vi "CLC_JIO_subUDC.vi"(5 "Mode":T1=enum."Tx", 8 "error in":errorcluster, 10 "ud att":i32) -> (0 "error out":errorcluster, 3 "standard output":string)   [LabVIEW 2023, in "CLC_JIO_FTDI.lvlib"]
uses:
  CLC_JIO_FTDI.lvlib
  CTL/Mode_tx1_rx2.ctl
panel:
  out "appended path":path
  out "standard error":string
  out "floder?":bool
  # "0:Tx\n1:Rx"
  # "0-255"
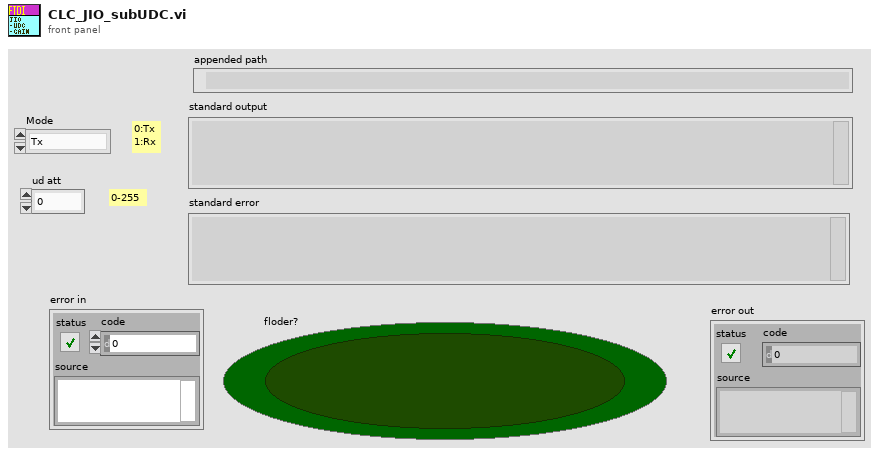
[diagram p1: front panel]
types:
  T1 = typedef "Mode_tx1_rx2.ctl" = enum16{"Standy", "Tx", "Rx"}
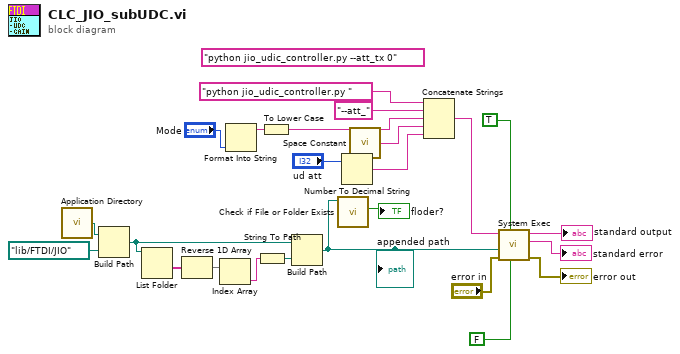
[diagram p0: block diagram]
diagram:
  (unwired) "python jio_udic_controller.py --att_tx 0" ("command line")
  n1 = call <vilib>:"Application Directory.vi"() -> ("Application Directory"=w16:path)
  n2 = Build Path(base path=w16, name or relative path=path "lib/FTDI/JIO") -> (appended path=w15:path)
  n3 = List Folder(path=w15) -> (folder names=w21:string[])  [unwired: 3 in, 3 out]
  n4 = Reverse 1D Array(array=w21) -> (reversed array=w20:string[])
  n5 = Index Array(array=w20) -> (element=w19:string)  [unwired: 1 in]
  n6 = Format Into String("Mode") -> (resulting string=w23:string)  [unwired: 3 in, 1 out]
  n7 = String To Path(string=w19) -> (path=w18:path)
  n8 = To Lower Case(string=w23) -> (all lower case string=w1:string)
  n9 = Build Path(base path=w15, name or relative path=w18) -> (appended path=w13:path)
  "appended path" <- w13
  n10 = call <vilib>:"Check if File or Folder Exists.vi"("path"=w13) -> ("file or folder exists?"=→"floder?":bool)  [unwired: 8 in, 2 out]
  n11 = Number To Decimal String(number="ud att") -> (decimal integer string=w3:string)  [unwired: 1 in]
  n12 = call <vilib>:"Space Constant.vi"() -> ("String"=w4:string)
  n13 = Concatenate Strings("python jio_udic_controller.py " ("string"), "--att_" ("string"), w1, w4, w3) -> (w2:string)
  n14 = call <vilib>:"System Exec.vi"("run minimized? (F)"=FALSE, "wait until completion? (T)"=TRUE, "error in (no error)"="error in", "working directory"=w13, "command line"=w2) -> ("error out"=→"error out":errorcluster, "standard error"=→"standard error":string, "standard output"=→"standard output":string)  [unwired: 3 in, 1 out]
